vi "Inventario Ventas.vi"(7 "Array":i32[](array[numeric]), 8 "error in (no error)":errorcluster, 9 "Ubicacion":string, 10 "Full pedido":string[][](array[string]), 11 "Inventario/ventas":bool) -> (0 "error out":errorcluster, 2 "Sobrantes":string[][](array[string]))   [LabVIEW 2018]
uses:
  Controles/Lista Modulos.ctl
  Comunicacion/Mensajes.lvlib
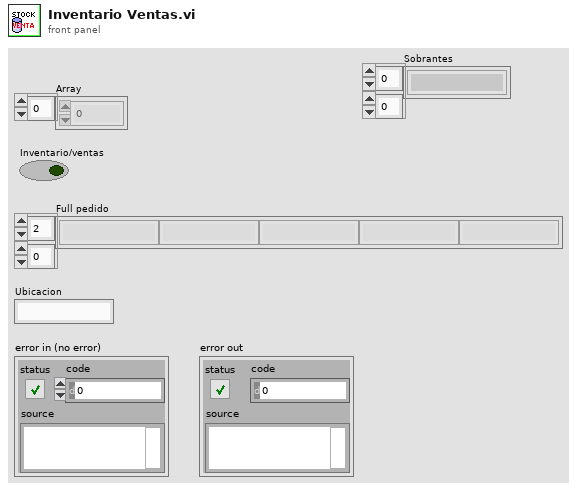
[diagram p1: front panel]
types:
  T1 = typedef "Lista Modulos.ctl" = enum16{"Math", "Error", "Front", "Database", "Nuevos items"}
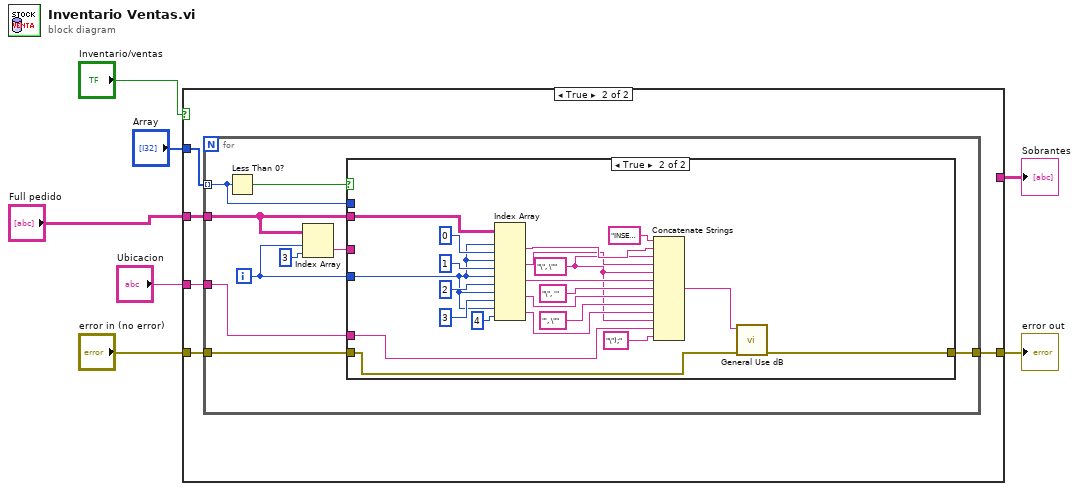
[diagram p0: block diagram]
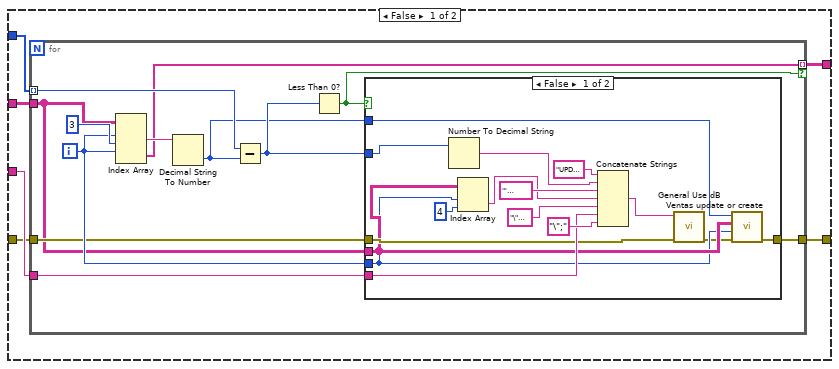
[diagram p2: hidden frame]
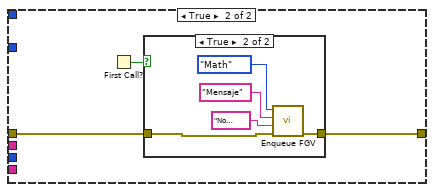
[diagram p3: hidden frame]
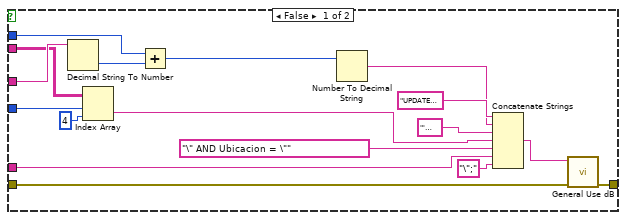
[diagram p5: hidden frame]
diagram:
  n1 = case shown="True" "Inventario/ventas" {
    tunnel: "Array" -> [w12 w55]
    tunnel: "Full pedido" -> [w13 w54]
    tunnel: "Ubicacion" -> [w11 w53]
    tunnel: "error in (no error)" -> [w10 w52]
    tunnel: [w9 w51] -> w7
    tunnel: [w8 _] -> w2
    frame False {
      n2 = for {
        tunnel: w13 -> [w15]
        tunnel: w12 -> [w24] mode=indexing
        tunnel: [w22] -> w8 mode=indexing if=w21
        tunnel: w11 -> [w18]
        tunnel: w10 -> [w17]
        tunnel: [w16] -> w9
        i -> [w19]
        n3 = Index Array(array=w15, index (row) #1=w19, index (col) #1=3 ("disabled index (col)"), index (row) #2=w19) -> (element #1=w23:string, element #2=w22:string[])  [unwired: 1 in]
        n4 = Decimal String To Number(string=w23) -> (number=w14:i32)  [unwired: 2 in, 1 out]
        n5 = Subtract(x=w24, y=w14) -> (x-y=w20:i32)
        n6 = Less Than 0?(x=w20) -> (x < 0?=w21:bool)
        n7 = case shown="False" w21 {
          tunnel: w20 -> [w35 _]
          tunnel: w15 -> [w30 _]
          tunnel: w19 -> [w29 _]
          tunnel: w18 -> [w32 _]
          tunnel: w17 -> [w31 w44]
          tunnel: [w26 w43] -> w16
          tunnel: w14 -> [w28 _]
          frame False {
            n8 = Number To Decimal String(number=w35) -> (decimal integer string=w40:string)  [unwired: 1 in]
            n9 = Index Array(array=w30, index (row)=w29, index (col)=4 ("disabled index (col)")) -> (element=w33:string)
            n10 = Concatenate Strings("UPDATE Inventario SET Cantidad = '" ("string"), w40, "' WHERE Codigo = \"" ("string"), w33, "\" AND Ubicacion = \"" ("string"), w32, "\";" ("string")) -> (w36:string)
            n11 = call "General Use dB.vi"("error in (no error)"=w31, "Query"=w36) -> ("error out"=w27:errorcluster)  [unwired: 8 in, 1 out]
            n12 = call "Ventas update or create.vi"("error in (no error)"=w27, "i"=w29, "Full pedido"=w30, "Vendidos"=w28) -> ("error out"=w26:errorcluster)  [unwired: 7 in]
          }
          frame True {
            n13 = First Call?() -> (First Call?: T/F=w42:bool)
            n14 = case shown="True" w42 {
              tunnel: w44 -> [w45 w50]
              tunnel: [w45 w49] -> w43
              frame False {
              }
              frame True {
                n15 = call "Enqueue FGV.vi"("error in (no error)"=w50, "Dato"="No suficientes en inventario" ("Mensaje"), "Mensaje"="Mensaje", "Modulo a obtener"=Lista_Modulos."Math") -> ("error out"=w49:errorcluster)  [unwired: 7 in]
              }
            }
          }
        }
      }
    }
    frame True {
      n16 = for {
        tunnel: w55 -> [w61] mode=indexing
        tunnel: w54 -> [w60]
        tunnel: w53 -> [w58]
        tunnel: w52 -> [w57]
        tunnel: [w56] -> w51
        i -> [w59]
        n17 = Less Than 0?(x=w61) -> (x < 0?=w63:bool)
        n18 = Index Array(array=w60, index (row)=w59, index (col)=3 ("disabled index (col)")) -> (element=w62:string)
        n19 = case shown="True" w63 {
          tunnel: w62 -> [w81 _]
          tunnel: w61 -> [w79 _]
          tunnel: w60 -> [w73 w101]
          tunnel: w59 -> [w74 w90]
          tunnel: w58 -> [w69 w86]
          tunnel: w57 -> [w67 w83]
          tunnel: [w66 w82] -> w56
          frame False {
            n20 = Decimal String To Number(string=w81) -> (number=w80:i32)  [unwired: 2 in, 1 out]
            n21 = Index Array(array=w73, index (row)=w74, index (col)=4 ("disabled index (col)")) -> (element=w71:string)
            n22 = Add(x=w79, y=w80) -> (x+y=w77:i32)
            n23 = Number To Decimal String(number=w77) -> (decimal integer string=w76:string)  [unwired: 1 in]
            n24 = Concatenate Strings("UPDATE Inventario SET Cantidad = '" ("string"), w76, "' WHERE Codigo = \"" ("string"), w71, "\" AND Ubicacion = \"" ("string"), w69, "\";" ("string")) -> (w65:string)
            n25 = call "General Use dB.vi"("error in (no error)"=w67, "Query"=w65) -> ("error out"=w66:errorcluster)  [unwired: 8 in, 1 out]
          }
          frame True {
            w87 = "\", \"" ("string")
            n26 = Index Array(array=w101, index (row) #1=w90, index (col) #1=0 ("disabled index (col)"), index (row) #2=w90, index (col) #2=1 ("disabled index (col)"), index (row) #3=w90, index (col) #3=2 ("disabled index (col)"), index (row) #4=w90, index (col) #4=3 ("disabled index (col)"), index (row) #5=w90, index (col) #5=4 ("disabled index (col)")) -> (element #1=w97:string, element #2=w96:string, element #3=w95:string, element #4=w92:string, element #5=w88:string)
            n27 = Concatenate Strings("INSERT INTO Inventario (Modelo,Color,Talla,Cantidad,Codigo,Ubicacion) VALUES (\" " ("string"), w97, w87, w96, w87, w95, "\", '" ("string"), w92, "', \"" ("string"), w88, w87, w86, "\");" ("string")) -> (w84:string)
            n28 = call "General Use dB.vi"("error in (no error)"=w83, "Query"=w84) -> ("error out"=w82:errorcluster)  [unwired: 8 in, 1 out]
          }
        }
      }
    }
  }
  "error out" <- w7
  "Sobrantes" <- w2
